vi "Calculadora.vi"() -> ()   [LabVIEW 2018]
uses:
  <vilib>/gmath/NI_Gmath.lvlib
panel:
  in  "RAD-DEG":enum32{"RADIANES", "GRADOS"}(radio)
  in  "Raizn":bool caption="/"
  in  "Raiz3":bool caption="/"
  in  "x!":bool caption="/"
  in  "1/x":bool caption="/"
  in  "^3":bool caption="/"
  in  "^2":bool caption="/"
  in  "logx":bool caption="/"
  in  "sqrt":bool caption="/"
  in  "ln":bool caption="/"
  in  "log":bool caption="/"
  in  "Ans":bool caption="/"
  in  "e":bool caption="/"
  in  "Pi":bool caption="/"
  in  "INV":bool caption="/"
  in  "tanh":bool caption="/"
  in  "cosh":bool caption="/"
  in  "sinh":bool caption="/"
  in  "tan":bool caption="/"
  in  "cos":bool caption="/"
  in  "sin":bool caption="/"
  in  "C":bool caption="/"
  in  "Bandera1":bool
  in  "DEL":bool caption="/"
  in  "Exp":bool caption="/"
  in  "^":bool caption="/"
  in  ")":bool caption="/"
  in  "(":bool caption="/"
  out "Last_Res":string
  in  "Bandera":bool
  in  "Igual":bool caption="="
  in  "Cluster":T1
  out "Display":string
  # "CALCULADORA REALIZADA POR:\nCARLOS HUGO OSORIO PATIÑO."
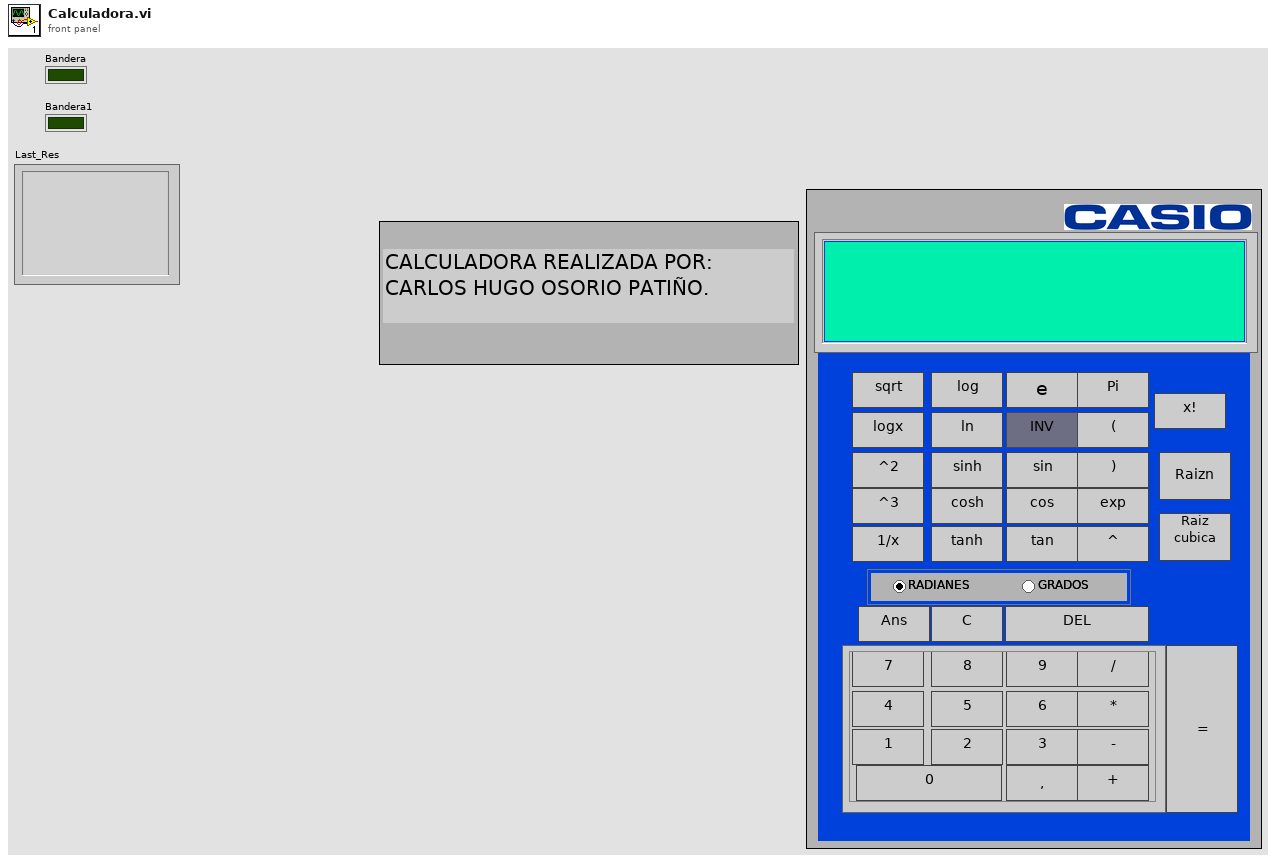
[diagram p1: front panel]
types:
  T1 = cluster{"1":bool, "2":bool, "3":bool, "4":bool, "5":bool, "6":bool, "7":bool, "8":bool, "9":bool, "0":bool, "coma":bool, "restar":bool, "multiplicar":bool, "dividir":bool, "sumar":bool}
  T2 = typedef "eventvkey.ctl" = enum16{"ASCII", "Enter", "Return", "Shift", "Ctrl", "Alt", "Cmd", "Opt", "Caps", "NumLock", "Clear", "Break", "Up", "Down", "Left", "Right", "Insert", "Delete", "Home", "End", "PageUp", "PageDown", "Escape", "Help", "Pause", "ScrollLock", "F1", "F2", "F3", "F4", "F5", "F6", "F7", "F8", "F9", "F10", "F11", "F12", "F13", "F14", "F15", "F16", "F17", "F18", "F19", "F20", "F21", "F22", "F23", "F24", "Play", "VolumeUp", "VolumeDown", "Mute", "Two Byte Char"}
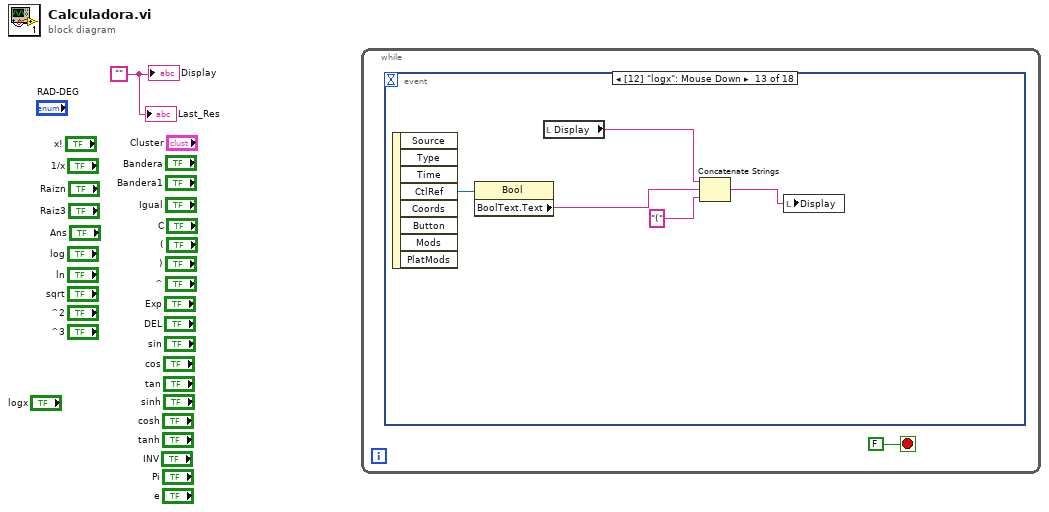
[diagram p0: block diagram]
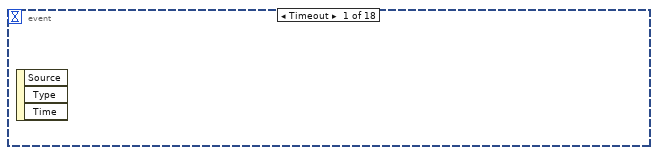
[diagram p2: hidden frame]
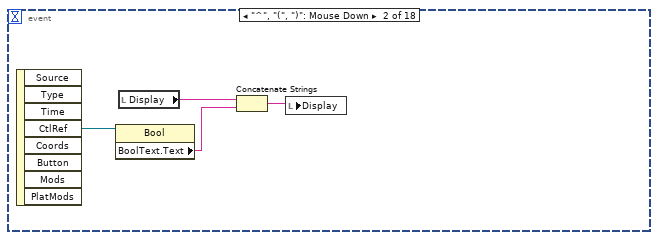
[diagram p3: hidden frame]
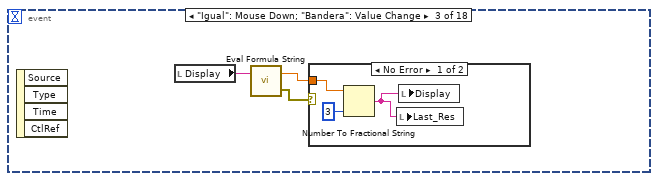
[diagram p4: hidden frame]
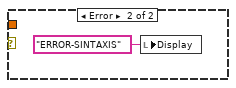
[diagram p5: hidden frame]
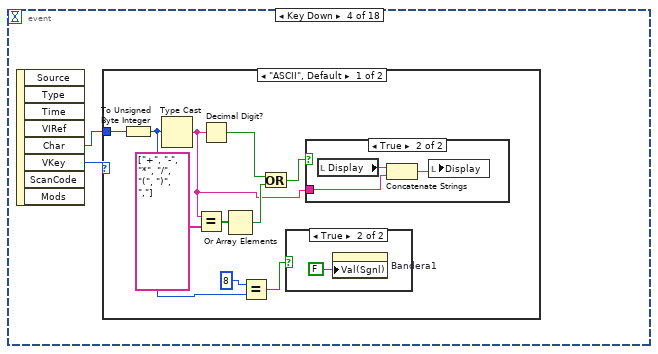
[diagram p6: hidden frame]
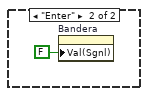
[diagram p9: hidden frame]
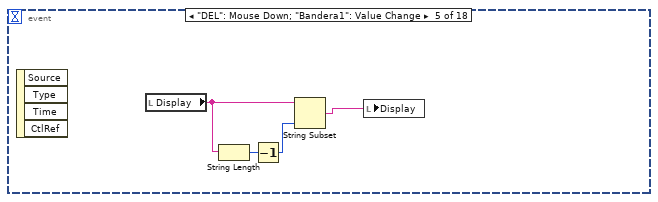
[diagram p10: hidden frame]
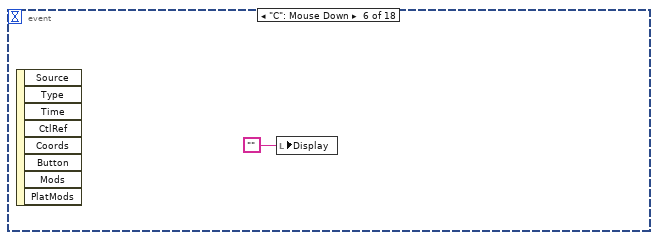
[diagram p11: hidden frame]
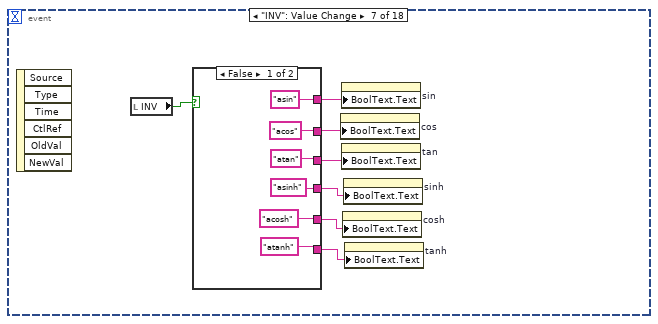
[diagram p12: hidden frame]
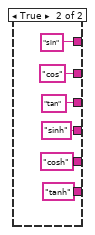
[diagram p13: hidden frame]
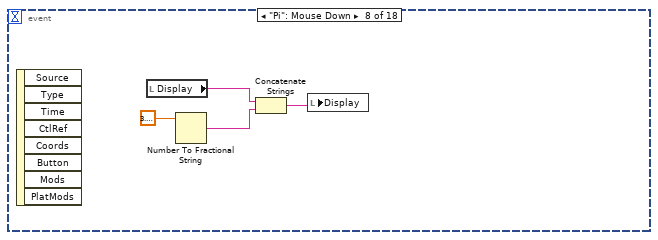
[diagram p14: hidden frame]
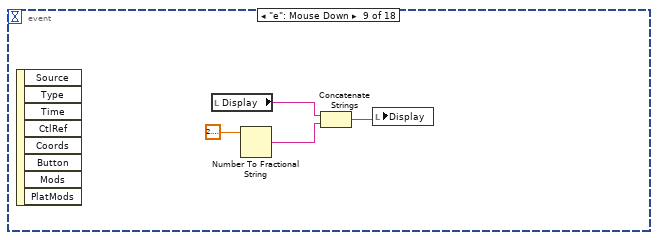
[diagram p15: hidden frame]
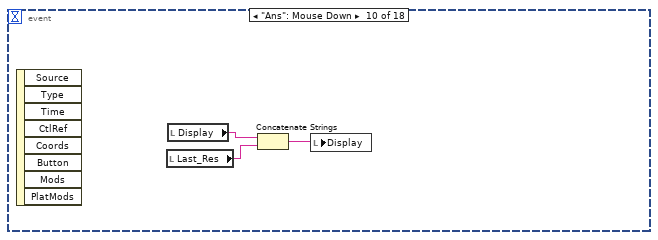
[diagram p16: hidden frame]
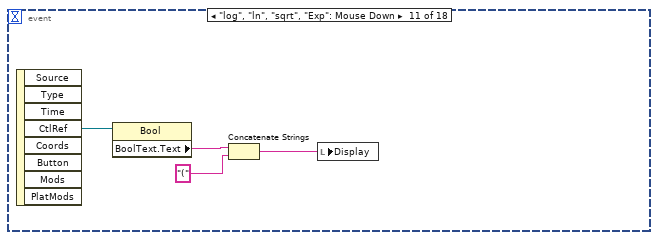
[diagram p17: hidden frame]
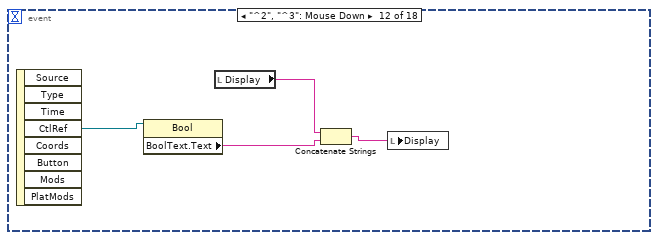
[diagram p18: hidden frame]
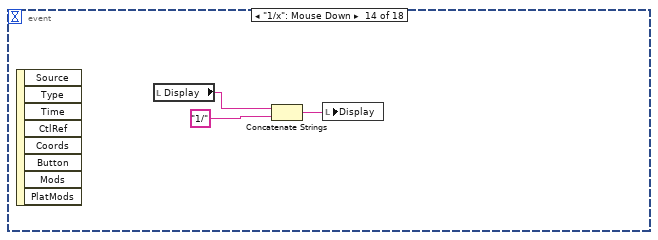
[diagram p19: hidden frame]
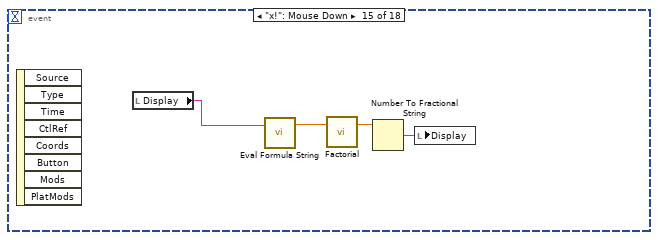
[diagram p20: hidden frame]
diagram:
  w1 = ""
  n1 = while {
    stop <- FALSE stop-if-true
    n2 = event shown="[12] \"logx\": Mouse Down" {
      selector: _ -> [_ _ _ _ _ _ _ _ _ _ _ _ _ _ _ _ _ _]
      dyn-events: _ -> [_ _ _ _ _ _ _ _ _ _ _ _ _ _ _ _ _ _]
      timeout: _ -> [_ _ _ _ _ _ _ _ _ _ _ _ _ _ _ _ _ _]
      event Timeout {
        n3 = event-data() -> ()  [unwired: 1 in, 3 out]
      }
      event "^", "Cluster.2", "Cluster.3", "Cluster.4", "Cluster.5", "Cluster.6", "Cluster.7", "Cluster.8", "Cluster.9", "Cluster.0", "Cluster.coma", "Cluster.restar", "Cluster.multiplicar", "Cluster.dividir", "Cluster.sumar", "(", ")", "Cluster.1": Mouse Down {
        n4 = event-data() -> ("CtlRef"=w4:refnum<vi>)  [unwired: 1 in, 7 out]
        n5 = property class="Bool"(reference=w4) -> ("BoolText.Text"=w3:string)  [unwired: 1 in, 2 out]
        n6 = local read "Display"() -> (w6:string)
        n7 = Concatenate Strings(w6, w3) -> (w5:string)
        n8 = local write "Display"(w5) -> ()
      }
      event "Igual": Mouse Down; "Bandera": Value Change {
        n9 = event-data() -> ()  [unwired: 1 in, 4 out]
        n10 = local read "Display"() -> (w7:string)
        n11 = call <vilib>:"Eval Formula String.vi"("formula"=w7) -> ("error out"=w8:errorcluster, "y value"=w9:dbl)  [unwired: 1 in]
        n12 = case shown="No Error" w8 {
          tunnel: w9 -> [w12 _]
          frame No Error {
            n13 = Number To Fractional String(number=w12, precision (6)=i16 3) -> (F-format string=w10:string)  [unwired: 2 in]
            n14 = local write "Last_Res"(w10) -> ()
            n15 = local write "Display"(w10) -> ()
          }
          frame Error {
            n16 = local write "Display"("ERROR-SINTAXIS" ("Display")) -> ()
          }
        }
      }
      event Key Down {
        n17 = event-data() -> ("Char"=w14:i16, "VKey"=w15:T2)  [unwired: 1 in, 6 out]
        n18 = case shown="\"ASCII\", Default" w15 {
          tunnel: w14 -> [w25 _]
          frame "ASCII", Default {
            n19 = To Unsigned Byte Integer(number=w25) -> (unsigned 8bit integer=w18:u8)
            n20 = Type Cast(x=w18) -> (*(type *) &x=w19:string)  [unwired: 1 in]
            n21 = Equal?(x=w19, y=string[] ["+", "-", "*", "/", "(", ")", ","]) -> (x = y?=w22:bool[])
            n22 = Decimal Digit?(1:w19) -> (0:w24:bool)
            n23 = Or Array Elements(Boolean array=w22) -> (logical OR=w21:bool)
            n24 = Equal?(x=u8 8, y=w18) -> (x = y?=w16:bool)
            n25 = Or(x=w24, y=w21) -> (x .or. y?=w20:bool)
            n26 = case shown="True" w16 {
              frame False {
              }
              frame True {
                n27 = property on="Bandera1" class="Bool (strict)"("Val(Sgnl)"=FALSE ("Value (Signaling)")) -> ()  [unwired: 2 in, 2 out]
              }
            }
            n28 = case shown="True" w20 {
              tunnel: w19 -> [_ w27]
              frame False {
              }
              frame True {
                n29 = local read "Display"() -> (w28:string)
                n30 = Concatenate Strings(w28, w27) -> (w29:string)
                n31 = local write "Display"(w29) -> ()
              }
            }
          }
          frame "Enter" {
            n32 = property on="Bandera" class="Bool (strict)"("Val(Sgnl)"=FALSE ("Value (Signaling)")) -> ()  [unwired: 2 in, 2 out]
          }
        }
      }
      event "DEL": Mouse Down; "Bandera1": Value Change {
        n33 = event-data() -> ()  [unwired: 1 in, 4 out]
        n34 = local read "Display"() -> (w34:string)
        n35 = String Length(string=w34) -> (length=w33:i32)
        n36 = Decrement(x=w33) -> (x-1=w32:i32)
        n37 = String Subset(string=w34, length (rest)=w32) -> (substring=w31:string)  [unwired: 1 in]
        n38 = local write "Display"(w31) -> ()
      }
      event "C": Mouse Down {
        n39 = event-data() -> ()  [unwired: 1 in, 8 out]
        n40 = local write "Display"("") -> ()
      }
      event "INV": Value Change {
        n41 = event-data() -> ()  [unwired: 1 in, 6 out]
        n42 = local read "INV"() -> (w42:bool)
        n43 = case shown="False" w42 {
          tunnel: ["asin" "sin"] -> w41
          tunnel: ["acos" "cos"] -> w40
          tunnel: ["atan" "tan"] -> w39
          tunnel: ["asinh" "sinh"] -> w38
          tunnel: ["acosh" "cosh"] -> w37
          tunnel: ["atanh" "tanh"] -> w36
          frame False {
          }
          frame True {
          }
        }
        n44 = property on="cos" class="Bool"("BoolText.Text"=w40) -> ()  [unwired: 2 in, 2 out]
        n45 = property on="sin" class="Bool"("BoolText.Text"=w41) -> ()  [unwired: 2 in, 2 out]
        n46 = property on="tan" class="Bool"("BoolText.Text"=w39) -> ()  [unwired: 2 in, 2 out]
        n47 = property on="cosh" class="Bool"("BoolText.Text"=w37) -> ()  [unwired: 2 in, 2 out]
        n48 = property on="sinh" class="Bool"("BoolText.Text"=w38) -> ()  [unwired: 2 in, 2 out]
        n49 = property on="tanh" class="Bool"("BoolText.Text"=w36) -> ()  [unwired: 2 in, 2 out]
      }
      event "Pi": Mouse Down {
        n50 = event-data() -> ()  [unwired: 1 in, 8 out]
        n51 = local read "Display"() -> (w56:string)
        n52 = Number To Fractional String(number=3.141592653589793) -> (F-format string=w57:string)  [unwired: 3 in]
        n53 = Concatenate Strings(w56, w57) -> (w55:string)
        n54 = local write "Display"(w55) -> ()
      }
      event "e": Mouse Down {
        n55 = event-data() -> ()  [unwired: 1 in, 8 out]
        n56 = local read "Display"() -> (w61:string)
        n57 = Number To Fractional String(number=2.718281828459045) -> (F-format string=w62:string)  [unwired: 3 in]
        n58 = Concatenate Strings(w61, w62) -> (w60:string)
        n59 = local write "Display"(w60) -> ()
      }
      event "Ans": Mouse Down {
        n60 = event-data() -> ()  [unwired: 1 in, 8 out]
        n61 = local read "Last_Res"() -> (w64:string)
        n62 = local read "Display"() -> (w65:string)
        n63 = Concatenate Strings(w65, w64) -> (w63:string)
        n64 = local write "Display"(w63) -> ()
      }
      event "log", "ln", "sqrt", "Exp": Mouse Down {
        n65 = event-data() -> ("CtlRef"=w69:refnum<vi>)  [unwired: 1 in, 7 out]
        n66 = property class="Bool"(reference=w69) -> ("BoolText.Text"=w68:string)  [unwired: 1 in, 2 out]
        n67 = Concatenate Strings(w68, "(") -> (w66:string)
        n68 = local write "Display"(w66) -> ()
      }
      event "^2", "^3": Mouse Down {
        n69 = event-data() -> ("CtlRef"=w73:refnum<vi>)  [unwired: 1 in, 7 out]
        n70 = property class="Bool"(reference=w73) -> ("BoolText.Text"=w71:string)  [unwired: 1 in, 2 out]
        n71 = local read "Display"() -> (w72:string)
        n72 = Concatenate Strings(w72, w71) -> (w70:string)
        n73 = local write "Display"(w70) -> ()
      }
      event "logx": Mouse Down {
        n74 = event-data() -> ("CtlRef"=w76:refnum<vi>)  [unwired: 1 in, 7 out]
        n75 = property class="Bool"(reference=w76) -> ("BoolText.Text"=w74:string)  [unwired: 1 in, 2 out]
        n76 = local read "Display"() -> (w78:string)
        n77 = Concatenate Strings(w78, w74, "(") -> (w77:string)
        n78 = local write "Display"(w77) -> ()
      }
      event "1/x": Mouse Down {
        n79 = event-data() -> ()  [unwired: 1 in, 8 out]
        n80 = local read "Display"() -> (w81:string)
        n81 = Concatenate Strings(w81, "1/" ("string")) -> (w79:string)
        n82 = local write "Display"(w79) -> ()
      }
      event "x!": Mouse Down {
        n83 = event-data() -> ()  [unwired: 1 in, 8 out]
        n84 = local read "Display"() -> (w83:string)
        n85 = call <vilib>:"Eval Formula String.vi"("formula"=w83) -> ("y value"=w85:dbl)  [unwired: 1 in, 1 out]
        n86 = call <vilib>:"Factorial.vi"("n"=w85) -> ("n!"=w84:dbl)  [unwired: 2 in]
        n87 = Number To Fractional String(number=w84) -> (F-format string=w82:string)  [unwired: 3 in]
        n88 = local write "Display"(w82) -> ()
      }
      event "Raiz3": Mouse Down {
        n89 = event-data() -> ()  [unwired: 1 in, 8 out]
        n90 = local read "Display"() -> (w91:string)
        n91 = call <vilib>:"Eval Formula String.vi"("formula"=w91) -> ("y value"=w88:dbl)  [unwired: 1 in, 1 out]
        n92 = Reciprocal(x=3.0) -> (1/x=w87:dbl)
        n93 = Power Of X(1:w88, 2:w87) -> (0:w86:dbl)
        n94 = Number To Fractional String(number=w86) -> (F-format string=w90:string)  [unwired: 3 in]
        n95 = local write "Display"(w90) -> ()
      }
      event "Raizn": Mouse Down {
        n96 = event-data() -> ()  [unwired: 1 in, 8 out]
        n97 = local read "Display"() -> (w93:string)
        n98 = Concatenate Strings(w93, "^(1/" ("string")) -> (w94:string)
        n99 = local write "Display"(w94) -> ()
      }
      event "sin", "cos", "tan", "sinh", "cosh", "tanh": Mouse Down {
        n100 = event-data() -> ("CtlRef"=w96:refnum<vi>)  [unwired: 1 in, 7 out]
        n101 = local read "INV"() -> (w95:bool)
        n102 = case shown="False" w95 {
          tunnel: w96 -> [w97 w113]
          frame False {
            n103 = property class="Bool"(reference=w97) -> ("BoolText.Text"=w99:string)  [unwired: 1 in, 2 out]
            n104 = local read "RAD-DEG"() -> (w100:enum32{"RADIANES", "GRADOS"})
            n105 = case shown="\"GRADOS\"" w100 {
              tunnel: w99 -> [w102 w106]
              tunnel: [w101 w108] -> w98
              frame "RADIANES", Default {
                n106 = local read "Display"() -> (w104:string)
                n107 = Concatenate Strings(w104, w102, "(" ("string")) -> (w101:string)
              }
              frame "GRADOS" {
                n108 = local read "Display"() -> (w109:string)
                n109 = Concatenate Strings(w109, "57,3*" ("string"), w106, "(" ("string")) -> (w108:string)
              }
            }
            n110 = local write "Display"(w98) -> ()
          }
          frame True {
            n111 = property class="Bool"(reference=w113) -> ("BoolText.Text"=w111:string)  [unwired: 1 in, 2 out]
            n112 = local read "RAD-DEG"() -> (w112:enum32{"RADIANES", "GRADOS"})
            n113 = case shown="\"GRADOS\"" w112 {
              tunnel: w111 -> [w115 w120]
              tunnel: [w114 w119] -> w110
              frame "RADIANES", Default {
                n114 = local read "Display"() -> (w117:string)
                n115 = Concatenate Strings(w117, w115, "(" ("string")) -> (w114:string)
              }
              frame "GRADOS" {
                n116 = local read "Display"() -> (w121:string)
                n117 = Concatenate Strings(w121, w120, "(0,017452*" ("string")) -> (w119:string)
              }
            }
            n118 = local write "Display"(w110) -> ()
          }
        }
      }
    }
  }
  "Display" <- w1
  "Last_Res" <- w1
